vi "Module Loop.vi"(8 "error in (no error)":errorcluster, 11 "GUI Helper in":refnum<class "GUI Helper.lvclass">) -> (0 "error out":errorcluster, 3 "GUI Helper out":refnum<class "GUI Helper.lvclass">)   [LabVIEW 2020, in "VolatusGUI.lvlib" / "GUI Helper.lvclass"]
uses:
  GUI Helper.lvclass
  C:/dev/lv20CE/relink/lv-volatus/Volatus/Module/Module.lvclass
  GUI Helper.lvclass/GUI Helper.ctl
  Volatus/Show GUI Options.ctl
  Volatus/Module/Module.lvclass/Module.ctl
  Volatus/MessageQ/MessageQ.lvclass/MessageQ.ctl
  Volatus/Module/Module.lvclass
  Visibility Message.ctl
  Bounds Message.ctl
  <vilib>/Utility/miscctls.llb/LVRectTypeDef.ctl
  Volatus/MessageQ/Send.vi
  Volatus/Module/Parent Q.vi
  <vilib>/Utility/error.llb/Error Cluster From Error Code.vi
  Volatus/Volatus.lvlib
panel:
  out "Parent ID":string
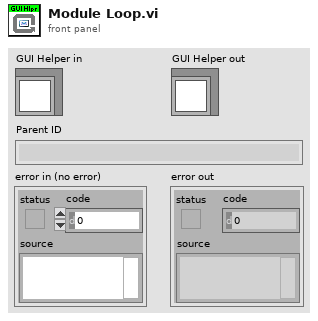
[diagram p1: front panel]
types:
  T1 = typedef "Volatus.lvlib/Show GUI Options.ctl" = cluster{"Show Core Module":bool}
  T2 = enum32{"Invalid", "Standard", "Closed", "Hidden", "Minimized", "Maximized"}
  T3 = typedef "VolatusGUI.lvlib/GUI Helper.lvclass/Visibility Message.ctl" = cluster{"Visible":bool}
  T4 = typedef "VolatusGUI.lvlib/GUI Helper.lvclass/Bounds Message.ctl" = cluster{"Bounds":T5}
  T5 = typedef "LVRectTypeDef.ctl" = cluster{"Left":i16, "Top":i16, "Right":i16, "Bottom":i16}
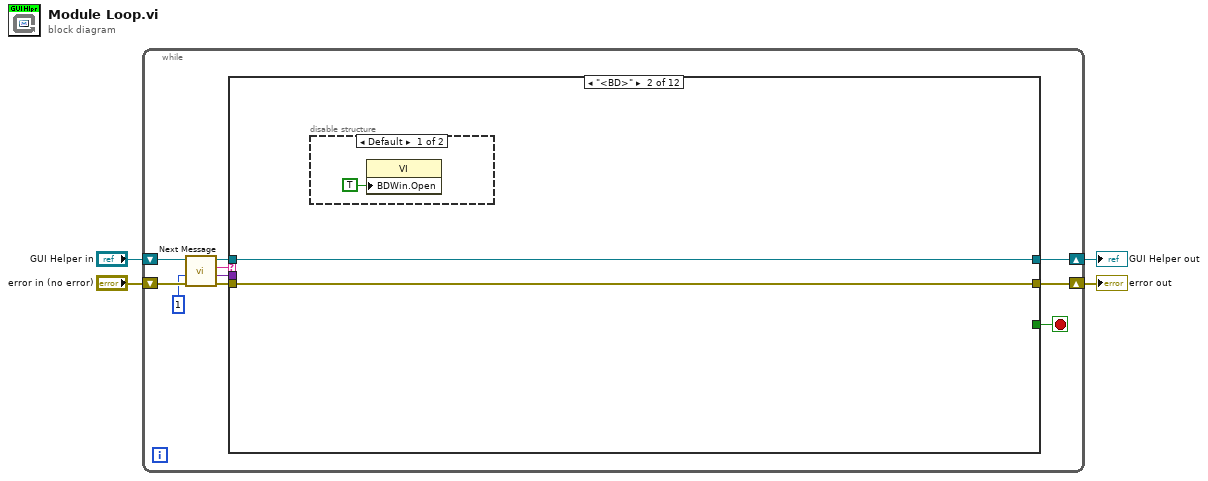
[diagram p0: block diagram]
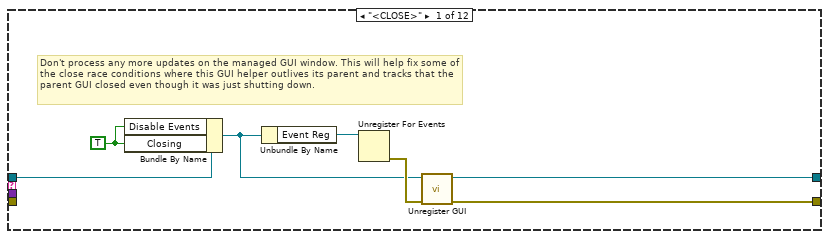
[diagram p2: hidden frame]
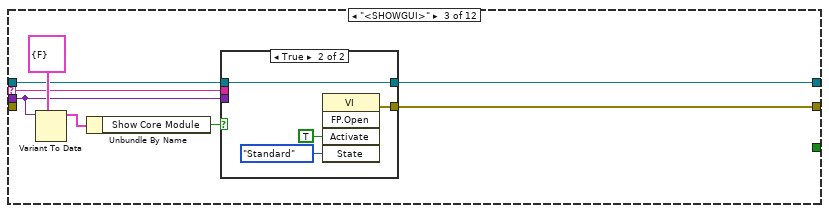
[diagram p4: hidden frame]
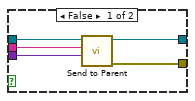
[diagram p5: hidden frame]
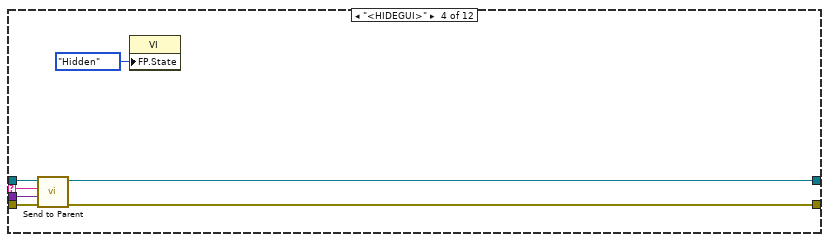
[diagram p6: hidden frame]
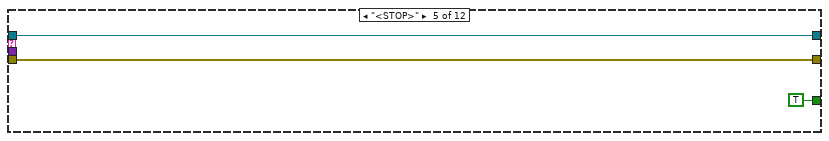
[diagram p7: hidden frame]
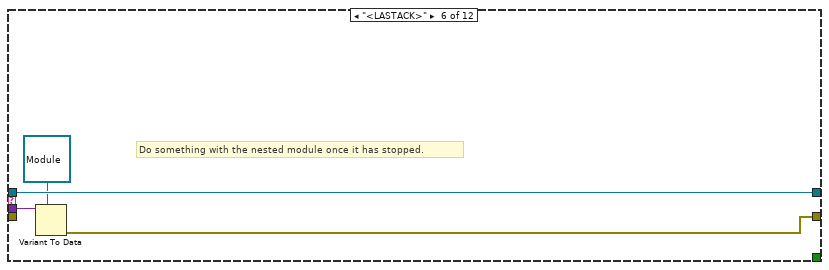
[diagram p8: hidden frame]
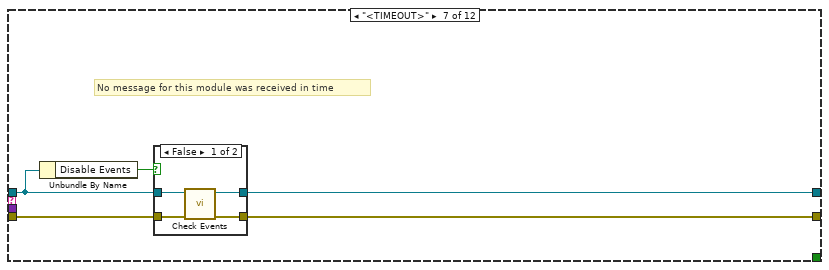
[diagram p9: hidden frame]
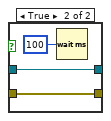
[diagram p10: hidden frame]
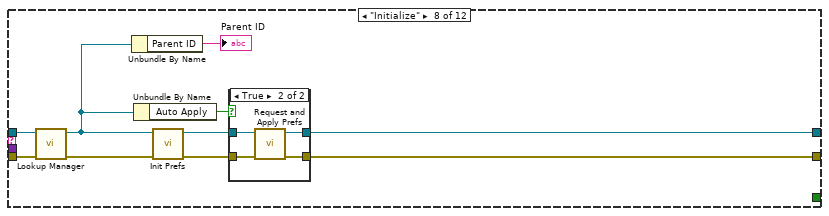
[diagram p11: hidden frame]
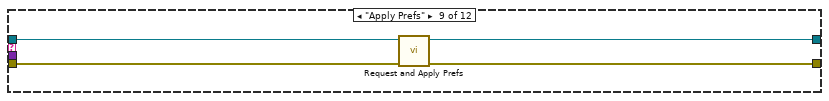
[diagram p13: hidden frame]
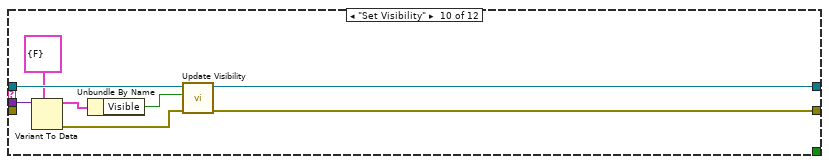
[diagram p14: hidden frame]
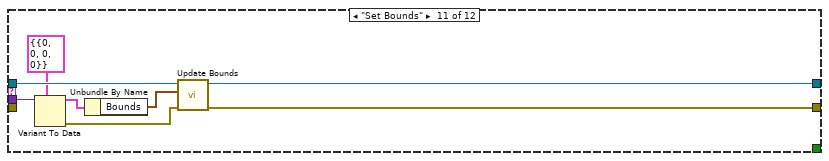
[diagram p15: hidden frame]
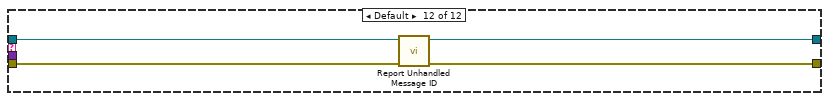
[diagram p16: hidden frame]
diagram:
  n1 = while {
    shift-right: [w9] -> w2
    shift-left: "GUI Helper in" -> [w14]
    shift-right: [w8] -> w3
    shift-left: "error in (no error)" -> [w13]
    stop <- w7 stop-if-true
    n2 = call "Next Message.vi"("error in (no error)"=w13, "Timeout ms (-1)"=1, "Module in"=w14) -> ("error out"=w12:errorcluster, "Data"=w6:variant, "ID"=w11:string, "Module out"=w10:refnum<class "GUI Helper.lvclass">)  [unwired: 5 in]
    n3 = case shown="\"<BD>\"" w11 {
      selector: w11 -> [_ _ w28 w43 _ _ _ _ _ _ _ _]
      tunnel: w12 -> [_ w22 _ w48 w50 _ w60 w77 w87 _ _ w107]
      tunnel: w10 -> [w20 w23 w30 w45 w51 w55 w56 w69 w85 w95 w103 w105]
      tunnel: [w16 w23 w26 w44 w51 w55 w58 w75 w84 w91 w99 w104] -> w9
      tunnel: [w15 w22 w25 w46 w50 w52 w59 w76 w86 w88 w96 w106] -> w8
      tunnel: [_ _ _ _ TRUE _ _ _ _ _ _ _] -> w7
      tunnel: w6 -> [_ _ w27 w42 _ w54 _ _ _ w94 w102 _]
      frame "<CLOSE>" {
        w19 = TRUE ("Closing")
        # "Don't process any more updates on the managed GUI window. This will help fix some of the close race conditions where this GUI helper outlives its parent and tracks that the parent GUI closed even though it was just shutting down."
        n4 = Bundle By Name(cluster=w20, "Disable Events"=w19, "Closing"=w19) -> (w18:refnum<class "GUI Helper.lvclass">)
        n5 = Unbundle By Name(w18) -> ("Event Reg"=w17:refnum<event-registration>)
        n6 = Unregister For Events(event registration refnum=w17) -> (error out=w21:errorcluster)  [unwired: 1 in]
        n7 = call "Unregister GUI.vi"("error in (no error)"=w21, "GUI Helper in"=w18) -> ("error out"=w15:errorcluster, "GUI Helper out"=w16:refnum<class "GUI Helper.lvclass">)  [unwired: 8 in]
      }
      frame "<BD>" {
        n8 = disable-structure shown="Default" {
          frame condition #0 (active) {
            n9 = property class="VI"("BDWin.Open"=TRUE ("Block Diagram Window:Open")) -> ()  [unwired: 2 in, 2 out]
          }
          frame condition #1 {
          }
        }
      }
      frame "<SHOWGUI>" {
        n10 = Variant To Data(type=T1 {"Show Core Module"=FALSE} ("Show GUI Options"), Variant=w27) -> (data=w29:T1)  [unwired: 1 in, 1 out]
        n11 = Unbundle By Name(w29) -> ("Show Core Module"=w31:bool)
        n12 = case shown="True" w31 {
          tunnel: w30 -> [w37 w39]
          tunnel: w28 -> [w36 _]
          tunnel: w27 -> [w35 _]
          tunnel: [w34 w39] -> w26
          tunnel: [w33 w38] -> w25
          frame False {
            n13 = call "Send to Parent.vi"("Data"=w35, "Message ID"=w36, "Module in"=w37) -> ("error out"=w33:errorcluster, "Module out"=w34:refnum<class "GUI Helper.lvclass">)  [unwired: 7 in]
          }
          frame True {
            n14 = invoke class="VI" method="FP.Open"("Activate"=TRUE ("Activate?"), "State"=T2."Standard") -> (error out=w38:errorcluster)  [unwired: 3 in, 4 out]
          }
        }
      }
      frame "<HIDEGUI>" {
        n15 = call "Send to Parent.vi"("error in (no error)"=w48, "Data"=w42, "Message ID"=w43, "Module in"=w45) -> ("error out"=w46:errorcluster, "Module out"=w44:refnum<class "GUI Helper.lvclass">)  [unwired: 6 in]
        n16 = property class="VI"("FP.State"=T2."Hidden" ("Front Panel Window:State")) -> ()  [unwired: 2 in, 2 out]
      }
      frame "<STOP>" {
      }
      frame "<LASTACK>" {
        # "Do something with the nested module once it has stopped."
        n17 = Variant To Data(type=refnum<class "Module.lvclass"> refnum ("Volatus:Module"), Variant=w54) -> (error out=w52:errorcluster)  [unwired: 1 in, 1 out]
      }
      frame "<TIMEOUT>" {
        # "No message for this module was received in time"
        n18 = Unbundle By Name(w56) -> ("Disable Events"=w57:bool)
        n19 = case shown="False" w57 {
          tunnel: w60 -> [w64 w66]
          tunnel: [w63 w66] -> w59
          tunnel: w56 -> [w62 w67]
          tunnel: [w61 w67] -> w58
          frame False {
            n20 = call "Check Events.vi"("error in (no error)"=w64, "GUI Helper in"=w62) -> ("error out"=w63:errorcluster, "GUI Helper out"=w61:refnum<class "GUI Helper.lvclass">)  [unwired: 8 in]
          }
          frame True {
            n21 = Wait (ms)(milliseconds to wait=u32 100) -> ()  [unwired: 1 out]
          }
        }
      }
      frame "Initialize" {
        n22 = call "Lookup Manager.vi"("error in (no error)"=w77, "GUI Helper in"=w69) -> ("error out"=w70:errorcluster, "GUI Helper out"=w68:refnum<class "GUI Helper.lvclass">)  [unwired: 8 in]
        n23 = Unbundle By Name(w68) -> ("Parent ID"=→"Parent ID":string)
        n24 = Unbundle By Name(w68) -> ("Auto Apply"=w74:bool)
        n25 = call "Init Prefs.vi"("error in (no error)"=w70, "GUI Helper in"=w68) -> ("error out"=w73:errorcluster, "GUI Helper out"=w72:refnum<class "GUI Helper.lvclass">)  [unwired: 8 in]
        n26 = case shown="True" w74 {
          tunnel: w73 -> [w78 w83]
          tunnel: [w78 w82] -> w76
          tunnel: [w79 w81] -> w75
          tunnel: w72 -> [w79 w80]
          frame False {
          }
          frame True {
            n27 = call "Request and Apply Prefs.vi"("error in (no error)"=w83, "GUI Helper in"=w80) -> ("error out"=w82:errorcluster, "GUI Helper out"=w81:refnum<class "GUI Helper.lvclass">)  [unwired: 8 in]
          }
        }
      }
      frame "Apply Prefs" {
        n28 = call "Request and Apply Prefs.vi"("error in (no error)"=w87, "GUI Helper in"=w85) -> ("error out"=w86:errorcluster, "GUI Helper out"=w84:refnum<class "GUI Helper.lvclass">)  [unwired: 8 in]
      }
      frame "Set Visibility" {
        n29 = Variant To Data(type=T3 {"Visible"=FALSE} ("Visibility Message"), Variant=w94) -> (data=w92:T3, error out=w89:errorcluster)  [unwired: 1 in]
        n30 = Unbundle By Name(w92) -> ("Visible"=w90:bool)
        n31 = call "Update Visibility.vi"("error in (no error)"=w89, "Visible"=w90, "GUI Helper in"=w95) -> ("error out"=w88:errorcluster, "GUI Helper out"=w91:refnum<class "GUI Helper.lvclass">)  [unwired: 7 in]
      }
      frame "Set Bounds" {
        n32 = Variant To Data(type=T4 {"Bounds"={"Left"=0, "Top"=0, "Right"=0, "Bottom"=0}} ("Bound Message"), Variant=w102) -> (data=w100:T4, error out=w97:errorcluster)  [unwired: 1 in]
        n33 = Unbundle By Name(w100) -> ("Bounds"=w98:T5)
        n34 = call "Update Bounds.vi"("error in (no error)"=w97, "Bounds"=w98, "GUI Helper in"=w103) -> ("error out"=w96:errorcluster, "GUI Helper out"=w99:refnum<class "GUI Helper.lvclass">)  [unwired: 7 in]
      }
      frame Default {
        n35 = call "Report Unhandled Message ID.vi"("error in (no error)"=w107, "Module in"=w105) -> ("error out"=w106:errorcluster, "Module out"=w104:refnum<class "GUI Helper.lvclass">)  [unwired: 8 in]
      }
    }
  }
  "error out" <- w3
  "GUI Helper out" <- w2
